vi "1_HelloWorld.vi"() -> ()   [LabVIEW 2015]
panel:
  out "String Display":string="Hello World!"
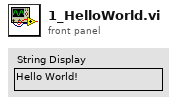
[diagram p1: front panel]
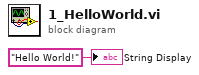
[diagram p0: block diagram]
diagram:
  "String Display" <- "Hello World!"
